vi "waveform_time_info.vi"() -> ()   [LabVIEW 2021]
panel:
  out "Waveform Graph":waveform(dbl)[](graph)
  out "Waveform Chart":waveform(dbl)[](graph)
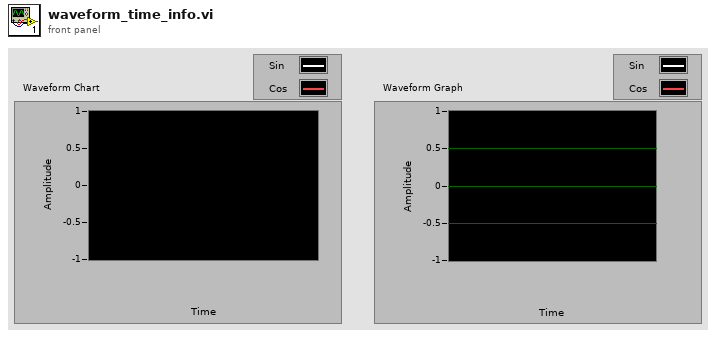
[diagram p1: front panel]
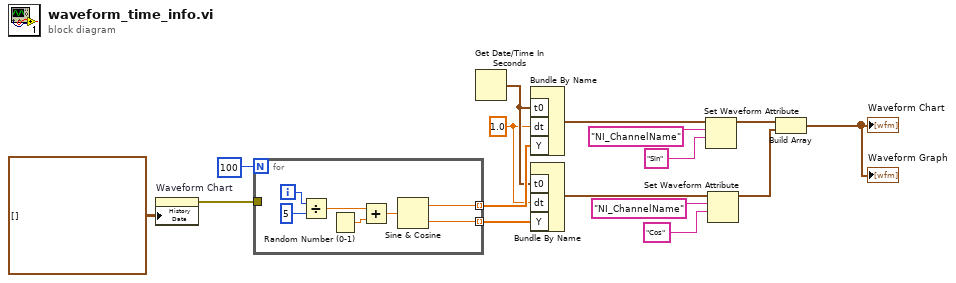
[diagram p0: block diagram]
diagram:
  w13 = 1.0 ("dt")
  n1 = property on="Waveform Chart" class="WFChart (strict)"("History Data"=waveform(dbl)[][] []) -> (error out=w1:errorcluster)  [unwired: 2 in, 1 out]
  n2 = for {
    N: 100 -> [_]
    tunnel: [w18] -> w15 mode=indexing
    tunnel: [w17] -> w12 mode=indexing
    tunnel: w1 -> [_]
    i -> [w23]
    n3 = Divide(x=w23, y=5) -> (x/y=w20:dbl)
    n4 = Random Number (0-1)() -> (number: 0 to 1=w21:dbl)
    n5 = Add(x=w20, y=w21) -> (x+y=w19:dbl)
    n6 = Sine & Cosine(0:w19) -> (1:w18:dbl, 2:w17:dbl)
  }
  n7 = Get Date/Time In Seconds() -> (seconds since 1Jan1904=w14:timestamp)
  n8 = Bundle By Name("t0"=w14, "dt"=w13, "Y"=w15) -> (w10:waveform(dbl))  [unwired: 1 in]
  n9 = Bundle By Name("t0"=w14, "dt"=w13, "Y"=w12) -> (w4:waveform(dbl))  [unwired: 1 in]
  n10 = Set Waveform Attribute(5:"Sin" ("name"), 6:"NI_ChannelName" ("name"), 7:w10) -> (3:w9:waveform(dbl))  [unwired: 1 in, 2 out]
  n11 = Set Waveform Attribute(5:"Cos" ("name"), 6:"NI_ChannelName" ("name"), 7:w4) -> (3:w3:waveform(dbl))  [unwired: 1 in, 2 out]
  n12 = Build Array "Build Array"(w9, w3) -> (→"Waveform Graph" →"Waveform Chart":waveform(dbl)[])
